vi "sleep_detection_criterion_total_immobility.vi"(3 "Deprivation\nparameters":T1={"Frame Row"=0, "Kstd"=40.0, "# Images for\nsleep detection"=10, "Kmean"=1.5, "Start time of sleep detection"=1000, 0, "Max deprivation length"=3600, "Max # TTL"=10000, "Delay detection start by x images after first detection"=0, "Minimum Interval between TTL pulses"=0, "Delay sleep detection\nby x detections"=9, "# Total immobility\n detections"=0.0, "Pause max # adjacent\nTTL"=0, "TTL x start\ntime deprivation\n"=0.0, "Max #\nadjacent TTL"=10000, " Ca2+\nmode"=0} {"?" items=["1", "2", "3", "4"]; "Frame Row" items=["1", "2", "3", "4"]}, 5 "Global image \nsubtraction array":dbl[](array[numeric]), 6 "Local image \nsubtraction array":dbl[](array[numeric])) -> (1 "Sleep detection":bool)   [LabVIEW 2011]
uses:
  <vilib>/Analysis/baseanly.llb/Std Deviation and Variance.vi
  <vilib>/Analysis/NI_AALBase.lvlib
panel:
  # "Sleep deprivation settings"
  # "Select deprivation animal"
  # "Deprive image in row"
  # "Deprive image in column"
  # "Sleep detection parameters"
  # "Sleep deprivation parameters"
  # "Delay deprivation start:"
  # "Pause deprivation (images):"
  # "Stop deprivation after:"
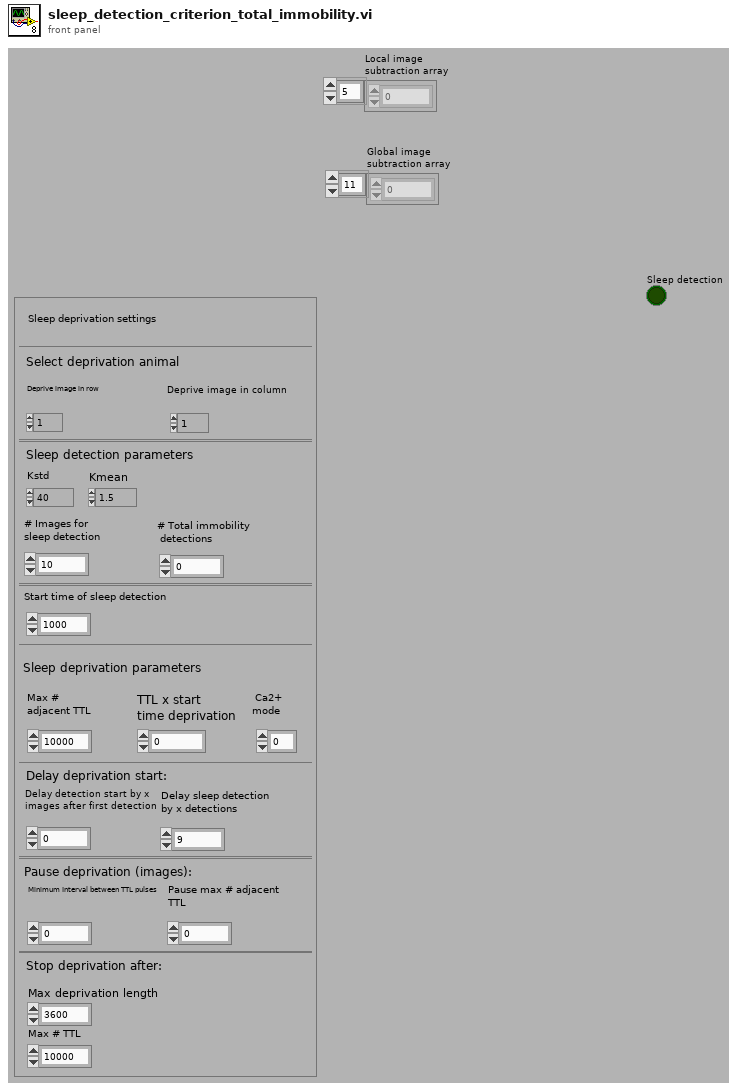
[diagram p1: front panel]
types:
  T1 = cluster{"Frame Row":u32, "Kstd":dbl, "# Images for\nsleep detection":i32, "Kmean":dbl, "Start time of sleep detection":i32, u32, "Max deprivation length":i32, "Max # TTL":i32, "Delay detection start by x images after first detection":i32, "Minimum Interval between TTL pulses":i32, "Delay sleep detection\nby x detections":i32, "# Total immobility\n detections":dbl, "Pause max # adjacent\nTTL":i32, "TTL x start\ntime deprivation\n":dbl, "Max #\nadjacent TTL":i32, " Ca2+\nmode":i32}
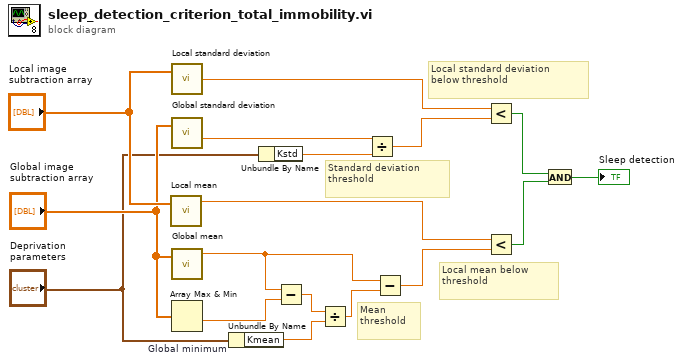
[diagram p0: block diagram]
diagram:
  # "Standard deviation\nthreshold"
  # "Mean \nthreshold"
  # "Local standard deviation\nbelow threshold"
  # "Local mean below\nthreshold"
  n1 = call "Local mean"("X"="Local image \nsubtraction array") -> ("mean"=w4:dbl)  [unwired: 1 in, 2 out]
  n2 = call "Local standard deviation"("X"="Local image \nsubtraction array") -> ("standard deviation"=w10:dbl)  [unwired: 1 in, 2 out]
  n3 = call "Global standard deviation"("X"="Global image \nsubtraction array") -> ("standard deviation"=w2:dbl)  [unwired: 1 in, 2 out]
  n4 = call "Global mean"("X"="Global image \nsubtraction array") -> ("mean"=w15:dbl)  [unwired: 1 in, 2 out]
  n5 = Array Max & Min "Global minimum"(array="Global image \nsubtraction array") -> (min value=w9:dbl)  [unwired: 3 out]
  n6 = Unbundle By Name("Deprivation\nparameters") -> ("Kmean"=w17:dbl)
  n7 = Unbundle By Name("Deprivation\nparameters") -> ("Kstd"=w6:dbl)
  n8 = Subtract(x=w15, y=w9) -> (x-y=w14:dbl)
  n9 = Divide(x=w14, y=w17) -> (x/y=w13:dbl)
  n10 = Divide(x=w2, y=w6) -> (x/y=w7:dbl)
  n11 = Subtract(x=w15, y=w13) -> (x-y=w8:dbl)
  n12 = Less?(x=w10, y=w7) -> (x < y?=w12:bool)
  n13 = Less?(x=w4, y=w8) -> (x < y?=w11:bool)
  n14 = And(x=w12, y=w11) -> (x .and. y?=→"Sleep detection":bool)
